vi "complex multiply by fxp_1.vi"(9 "input valid":bool, 10 "amp":fxp<+/-,18,1> format="%#_18g", 11 "IQ data":T1) -> (2 "data valid":bool, 3 "output cluster":T1)   [LabVIEW 2021]
uses:
  <instrlib>/_niInstr/DSP/v1/Shared/Public/IQ Data.ctl
  <vilib>/rvi/FXPMathLib/FxpMul/XNode/nifxpmath_Multiplier.xnode
  <vilib>/rvi/FXPMathLib/sim/FxpSim.dll
  <instrlib>/_niInstr/DSP/v1/Shared/niInstr DSP v1 Shared.lvlib
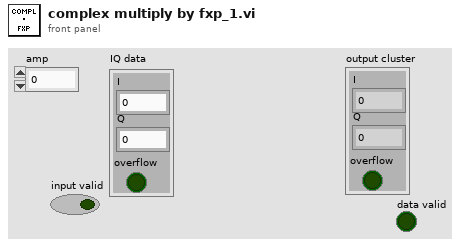
[diagram p1: front panel]
types:
  T1 = typedef "niInstr DSP v1 Shared.lvlib/IQ Data.ctl" = cluster{"I":fxp<+/-,18,1>, "Q":fxp<+/-,18,1>, "overflow":bool}
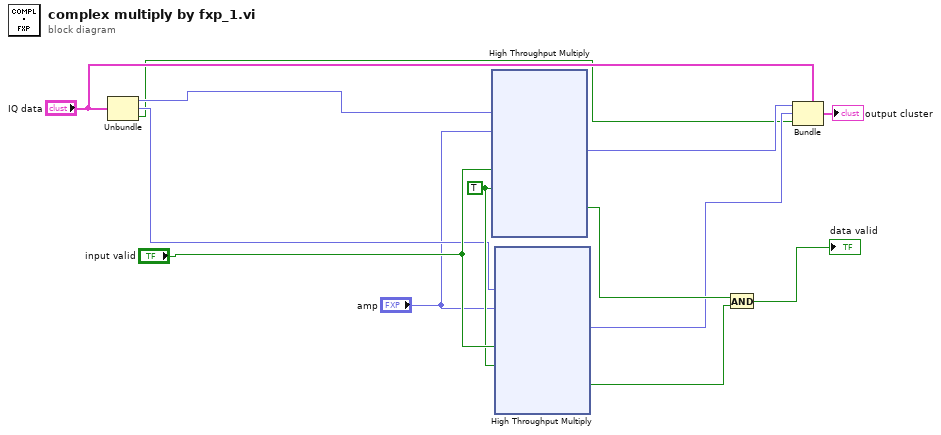
[diagram p0: block diagram]
diagram:
  w12 = TRUE ("ready for output (T)")
  n1 = Unbundle("IQ data") -> ("I"=w8:fxp<+/-,18,1>, "Q"=w7:fxp<+/-,18,1>, "overflow"=w2:bool)
  n2 = xnode ("High Throughput Multiply")("x"=w8, "y"="amp", "input valid"="input valid", "ready for output (T)"=w12) -> ("x*y"=w4:fxp<+/-,18,1>, "output valid"=w11:bool)  [unwired: 1 out]
  n3 = xnode ("High Throughput Multiply")("x"=w7, "y"="amp", "input valid"="input valid", "ready for output (T)"=w12) -> ("x*y"=w3:fxp<+/-,18,1>, "output valid"=w10:bool)  [unwired: 1 out]
  n4 = And(x=w11, y=w10) -> (x .and. y?=→"data valid":bool)
  n5 = Bundle(cluster="IQ data", "I"=w4, "Q"=w3, "overflow"=w2) -> (→"output cluster":T1)
